vi "Top (FPGA)-2-port.vi"() -> ()   [LabVIEW 2023, in "PXIe-7903 Aurora Example.lvlib"]
uses:
  PXIe-7903 Aurora Example.lvlib
  <vilib>/Platform/TimedLoop/XDataNode/wakeup.ctl
  <vilib>/Platform/TimedLoop/XDataNode/XDNodeRunTimeDep.lvlib
  <vilib>/Platform/TimedLoop/XDataNode/nitl_modes.ctl
  <vilib>/Platform/TimedLoop/XDataNode/timing_clust.ctl
  <vilib>/Platform/TimedLoop/XDataNode/XDataNode.xnode
  Program Files/NI/LVAddons/niidl/1/instr.lib/_niInstr/FIFO Register Bus/v1/FPGA/niInstr FIFO Register Bus v1 FPGA.lvclass
  Program Files/NI/LVAddons/niidl/1/instr.lib/_niInstr/Instruction Framework/v1/FPGA/Top Level Bus/Register Configuration/Register Configuration.lvclass
  Program Files/NI/LVAddons/niidl/1/instr.lib/_niInstr/Instruction Framework/v1/FPGA/Collection Builder/Collection Builder.lvclass
  Program Files/NI/LVAddons/niidl/1/instr.lib/_niInstr/Instruction Framework/v1/FPGA/Collection Builder/Parent Metadata.ctl
  Program Files/NI/LVAddons/niidl/1/instr.lib/_niInstr/Instruction Framework/v1/FPGA/Collection Builder/niInstr Address Space Collection Builder v1 FPGA.lvlib
  <vilib>/eio/EIONode/EIONode.xnode
  Utilities/FPGA/Aurora64b66b Utilities FPGA.lvlib
  Program Files/NI/LVAddons/niidl/1/instr.lib/_niInstr/Basic Elements/v1/FPGA/niInstr Basic Elements v1 FPGA.lvlib
  <vilib>/rvi/eio/common/nirviEmuTemplateMethod_errors.vi
  Program Files/NI/LVAddons/niidl/1/instr.lib/_niInstr/Aurora64b66b/v1/FPGA/Buffered/Aurora64b66b Buffered.lvclass
  C:/dev/github5/flexrio-custom/targets/pxie-7903/docs/Examples/AuroraCustom_LV2023/C/Program Files/NI/LVAddons/niidl/1/instr.lib/_niInstr/Instruction Framework/v1/FPGA/Interfaces/Instruction Producer/Instruction Producer.lvclass
  C:/dev/github5/flexrio-custom/targets/pxie-7903/docs/Examples/AuroraCustom_LV2023/C/Program Files/NI/LVAddons/niidl/1/instr.lib/_niInstr/FIFO Register Bus/v1/FPGA/niInstr FIFO Register Bus v1 FPGA.lvclass
panel:
  in  "port 1 enable":bool
  in  "port 0 enable":bool
  in  "port 1 rx throttle":u16
  out "port 1 mismatch count":u64
  out "port 0 mismatch count":u64
  in  "port 0 rx throttle":u16
  in  "tb reset":bool
  out "flexrio.module.io error 0":i32
  out "flexrio.module.io ready 0":bool
  in  "fifo reg bus ctrl 0":u32
  out "fifo reg bus status 0":u32
  out "fifo reg bus data 0":u64
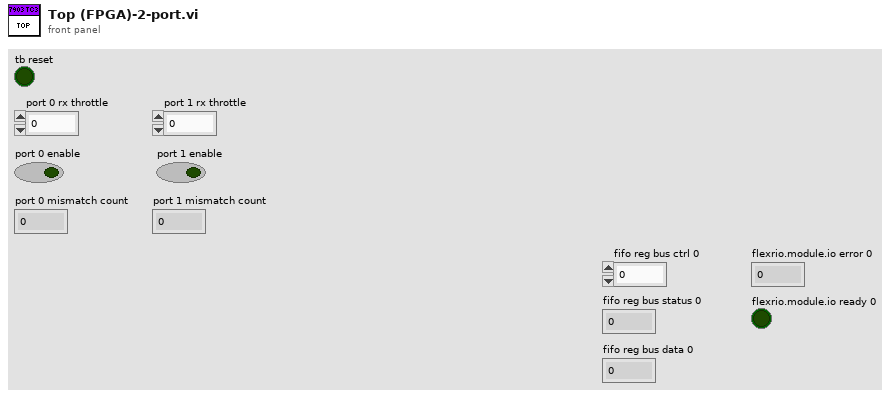
[diagram p1: front panel]
types:
  T1 = typedef "niInstr Address Space Collection Builder v1 FPGA.lvlib/Parent Metadata.ctl" = cluster{"UID":u16, "version":u16, "oldest compatible version":u16}
  T2 = typedef "XDNodeRunTimeDep.lvlib/timing_clust.ctl" = cluster{"Expected End [f-1]":u64, "Actual End [f-1]":u64, "Finished Late? [f-1]":bool, "Expected End [i-1]":u64, "Actual End [i-1]":u64, "Finished Late? [i-1]":bool, "Expected Start [i]":u64, "Actual Start [i]":u64, "Expected Start [f]":u64, "Actual Start [f]":u64, "Source Name":string, "Structure Name":string, "Period":i64, "Deadline":i64, "Offset":i64, "Start":i64, "Priority":i32, "Timeout":i32, "Mode":T3, "Wakeup Reason":T4, "Error":errorcluster, "Source Type":string, "Secondary Source Type":string, "Global End Time":u64, "Global Start Time":u64, "Frame Duration":u64, "Iteration Duration":u64, "Assigned CPU":i32, "I/O Scan Engine Mode":u32}
  T3 = typedef "XDNodeRunTimeDep.lvlib/nitl_modes.ctl" = enum32{"No Change", "Process missed periods, maintain original phase", "Discard missed periods, maintain original phase", "Process missed periods, ignore original phase", "Discard missed periods, ignore original phase"}
  T4 = typedef "XDNodeRunTimeDep.lvlib/wakeup.ctl" = enum32{"Normal", "Aborted", "Asynchronous wakeup", "Timing source error", "Timed loop error", "Timeout"}
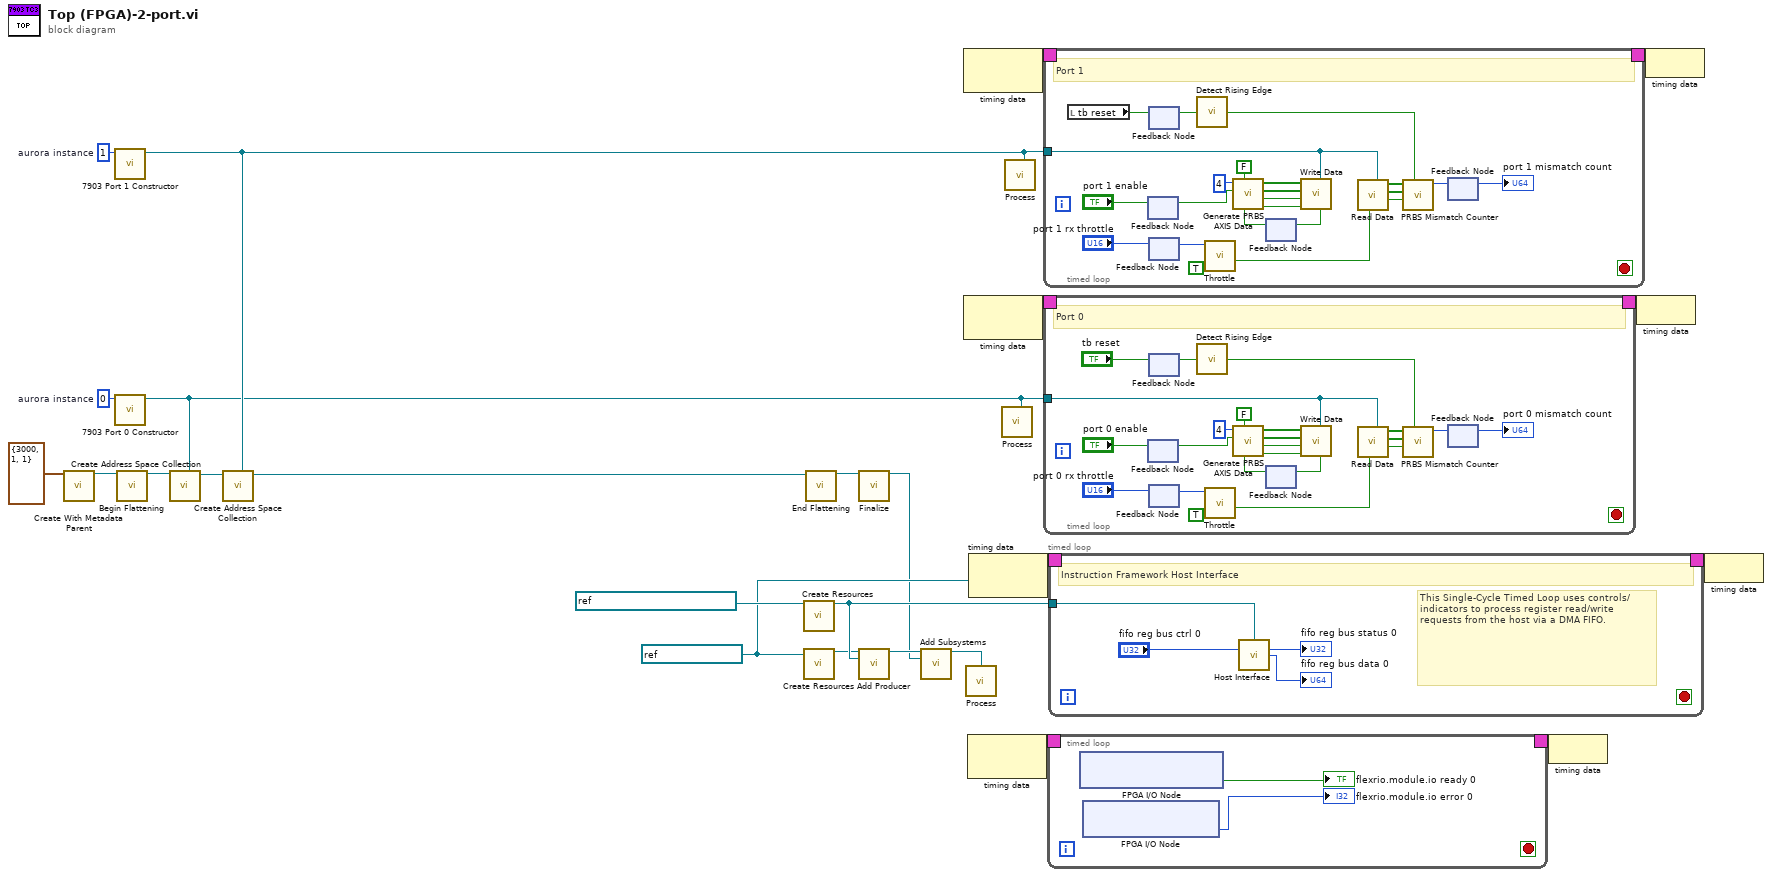
[diagram p0: block diagram]
diagram:
  w8 = u8 1  # aurora instance
  w9 = u8 0  # aurora instance
  w20 = refnum<k21> "80 MHz Clock" ("Source Name")
  n1 = call "Create With Metadata Parent.vi"("parent metadata"=T1 {"UID"=3000, "version"=1, "oldest compatible version"=1}) -> ("collection builder"=w19:refnum<class "Collection Builder.lvclass">)  [unwired: 14 in]
  n2 = call "7903 Port 1 Constructor.vi"("aurora instance (0)"=w8) -> ("aurora64b66b buffered"=w3:refnum<class "Aurora64b66b Buffered.lvclass">)  [unwired: 10 in]
  n3 = call "7903 Port 0 Constructor.vi"("aurora instance (0)"=w9) -> ("aurora64b66b buffered"=w2:refnum<class "Aurora64b66b Buffered.lvclass">)  [unwired: 10 in]
  n4 = call "Begin Flattening.vi"("collection builder in"=w19) -> ("collection builder out"=w13:refnum<class "Collection Builder.lvclass">)  [unwired: 14 in]
  n5 = call-dynamic "Create Address Space Collection.vi"("aurora64b66b basic"=w2, "collection builder in"=w13) -> ("collection builder out"=w10:refnum<class "Collection Builder.lvclass">)  [unwired: 9 in]
  n6 = call-dynamic "Create Address Space Collection.vi"("aurora64b66b basic"=w3, "collection builder in"=w10) -> ("collection builder out"=w1:refnum<class "Collection Builder.lvclass">)  [unwired: 9 in]
  n7 = call "Create Resources.vi"("instruction fifo"=refnum<k21> "reg.host instruction fifo 0" ("FIFO")) -> ("fifo register bus"=w22:refnum<class "niInstr FIFO Register Bus v1 FPGA.lvclass">)  [unwired: 14 in]
  n8 = call "Create Resources.vi"("register clock"=w20) -> ("register configuration"=w21:refnum<class "Register Configuration.lvclass">)  [unwired: 14 in]
  n9 = call "End Flattening.vi"("collection builder in"=w1) -> ("collection builder out"=w18:refnum<class "Collection Builder.lvclass">)  [unwired: 14 in]
  n10 = call "Finalize.vi"("collection builder in"=w18) -> ("address space collection"=w14:refnum<class "Address Space Collection.lvclass">)  [unwired: 14 in]
  n11 = call-dynamic "Add Producer.vi"("register configuration in"=w21, "instruction producer"=w22) -> ("register configuration out"=w16:refnum<class "Register Configuration.lvclass">)  [unwired: 13 in]
  n12 = call-dynamic "Add Subsystems.vi"("register configuration in"=w16, "subsystems"=w14) -> ("register configuration out"=w15:refnum<class "Register Configuration.lvclass">)  [unwired: 13 in]
  n13 = node-c288() -> (w5:T2)  [unwired: 1 in]
  n14 = node-c288() -> (w7:T2)  [unwired: 1 in]
  n15 = call-dynamic "Process.vi"("register configuration"=w15) -> ()  [unwired: 15 in]
  n16 = node-c288() -> (w12:T2)  [unwired: 1 in]
  n17 = node-c288(w20) -> (w25:T2)
  n18 = call-dynamic "Process.vi"("aurora64b66b buffered"=w2) -> ()  [unwired: 11 in]
  n19 = call-dynamic "Process.vi"("aurora64b66b buffered"=w3) -> ()  [unwired: 11 in]
  n20 = timed-loop {
    timing: w5 -> [_]
    timing-out: [_] -> w4
    tunnel: w3 -> [w31]
    stop <- _ stop-if-true
    # "Port 1"
    n21 = local read "tb reset"() -> (w29:bool)
    n22 = feedback #1() -> (w26:bool)  [unwired: 1 in]
    n23 = feedback-in #1("port 1 enable") -> ()
    n24 = feedback-in #2(w29) -> ()
    n25 = feedback #2() -> (w32:bool)  [unwired: 1 in]
    n26 = feedback #3() -> (w34:u16)  [unwired: 1 in]
    n27 = feedback-in #3("port 1 rx throttle") -> ()
    n28 = call "Detect Rising Edge.vi"("signal"=w32) -> ("edge detected"=w46:bool)  [unwired: 14 in]
    n29 = call "Throttle.vi"("request data"=TRUE ("Request Data"), "throttle"=w34) -> ("throttled request"=w39:bool)  [unwired: 9 in]
    n30 = feedback #4() -> (w44:bool)  [unwired: 1 in]
    n31 = call "Generate PRBS AXIS Data.vi"("ready for output"=w44, "reset"=FALSE, "enable"=w26, "number of lanes"=u8 4) -> ("tlast"=w40:bool, "tvalid"=w41:bool, "tkeep"=w42:bool[], "tdata"=w43:bool[])  [unwired: 4 in]
    n32 = call-dynamic "Write Data.vi"("aurora64b66b buffered"=w31, "tlast"=w40, "input valid"=w41, "tkeep"=w42, "tdata"=w43) -> ("ready for input"=w45:bool)  [unwired: 6 in]
    n33 = feedback-in #4(w45) -> ()
    n34 = call-dynamic "Read Data.vi"("aurora64b66b buffered"=w31, "ready for output"=w39) -> ("output valid"=w36:bool, "tkeep"=w37:bool[], "tdata"=w38:bool[])  [unwired: 6 in, 1 out]
    n35 = call "PRBS Mismatch Counter.vi"("reset mismatch count"=w46, "input valid"=w36, "tkeep"=w37, "data in"=w38) -> ("mismatch count"=w47:u64)  [unwired: 7 in]
    n36 = feedback-in #5(w47) -> ()
    n37 = feedback #5() -> (→"port 1 mismatch count":u64)  [unwired: 1 in]
  }
  n38 = timed-loop {
    timing: w7 -> [_]
    timing-out: [_] -> w6
    tunnel: w2 -> [w55]
    stop <- _ stop-if-true
    # "Port 0"
    n39 = feedback #6() -> (w51:bool)  [unwired: 1 in]
    n40 = feedback-in #6("port 0 enable") -> ()
    n41 = feedback-in #7("tb reset") -> ()
    n42 = feedback #7() -> (w56:bool)  [unwired: 1 in]
    n43 = feedback #8() -> (w59:u16)  [unwired: 1 in]
    n44 = feedback-in #8("port 0 rx throttle") -> ()
    n45 = call "Detect Rising Edge.vi"("signal"=w56) -> ("edge detected"=w71:bool)  [unwired: 14 in]
    n46 = call "Throttle.vi"("request data"=TRUE ("Request Data"), "throttle"=w59) -> ("throttled request"=w64:bool)  [unwired: 9 in]
    n47 = feedback #9() -> (w69:bool)  [unwired: 1 in]
    n48 = call "Generate PRBS AXIS Data.vi"("ready for output"=w69, "reset"=FALSE, "enable"=w51, "number of lanes"=u8 4) -> ("tlast"=w65:bool, "tvalid"=w66:bool, "tkeep"=w67:bool[], "tdata"=w68:bool[])  [unwired: 4 in]
    n49 = call-dynamic "Write Data.vi"("aurora64b66b buffered"=w55, "tlast"=w65, "input valid"=w66, "tkeep"=w67, "tdata"=w68) -> ("ready for input"=w70:bool)  [unwired: 6 in]
    n50 = feedback-in #9(w70) -> ()
    n51 = call-dynamic "Read Data.vi"("aurora64b66b buffered"=w55, "ready for output"=w64) -> ("output valid"=w61:bool, "tkeep"=w62:bool[], "tdata"=w63:bool[])  [unwired: 6 in, 1 out]
    n52 = call "PRBS Mismatch Counter.vi"("reset mismatch count"=w71, "input valid"=w61, "tkeep"=w62, "data in"=w63) -> ("mismatch count"=w72:u64)  [unwired: 7 in]
    n53 = feedback-in #10(w72) -> ()
    n54 = feedback #10() -> (→"port 0 mismatch count":u64)  [unwired: 1 in]
  }
  n55 = timed-loop {
    timing: w12 -> [_]
    timing-out: [_] -> w11
    stop <- _ stop-if-true
    n56 = xnode "FPGA I/O Node"() -> ("IO Socket.IO Ready"=→"flexrio.module.io ready 0":bool)  [unwired: 1 in, 1 out]
    n57 = xnode "FPGA I/O Node"() -> ("IO Socket.IO Error"=→"flexrio.module.io error 0":i32)  [unwired: 1 in, 1 out]
  }
  n58 = timed-loop {
    timing: w25 -> [_]
    timing-out: [_] -> w24
    tunnel: w22 -> [w80]
    stop <- _ stop-if-true
    # "This Single-Cycle Timed Loop uses controls/indicators to process register read/write requests from the host via a DMA FIFO."
    # "Instruction Framework Host Interface"
    n59 = call "Host Interface.vi"("fifo register bus"=w80, "fifo reg bus ctrl 0"="fifo reg bus ctrl 0") -> ("fifo reg bus status 0"=→"fifo reg bus status 0":u32, "fifo reg bus data 0"=→"fifo reg bus data 0":u64)  [unwired: 12 in]
  }
  n60 = node-c288(w11) -> ()
  n61 = node-c288(w6) -> ()
  n62 = node-c288(w4) -> ()
  n63 = node-c288(w24) -> ()
